vi "Test web service.vi"() -> ()   [LabVIEW 2012]
uses:
  Library/Shot data.ctl
panel:
  in  "Shot data":T1={"Shot number"=33, "Time"=timestamp(3410450400.259543 s since 1904-01-01), "Magnet ID"="sdqwde", "User"="sAXWCD", "Cell number"=1, "Requested field"=65.0, "Field direction"="UP", "Number of bank frames"=8, "Crowbar resistance, mOhm"=25.0, "Magnet resistance, mOhm"=35.0, "Charger voltage, kV"=9.0, "Frame voltage, kV"=10.0}
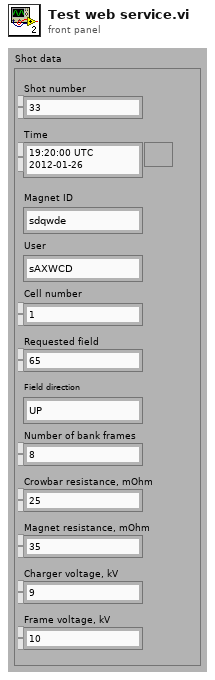
[diagram p1: front panel]
types:
  T1 = typedef "Shot data.ctl" = cluster{"Shot number":i32, "Time":timestamp, "Magnet ID":string, "User":string, "Cell number":i32, "Requested field":dbl, "Field direction":string, "Number of bank frames":i32, "Crowbar resistance, mOhm":dbl, "Magnet resistance, mOhm":dbl, "Charger voltage, kV":dbl, "Frame voltage, kV":dbl}
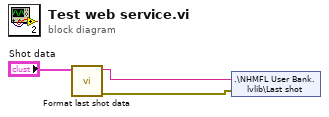
[diagram p0: block diagram]
diagram:
  n1 = call "Format last shot data.vi"("Shot data"="Shot data") -> ("error out"=w2:errorcluster, "Formated shot data"=w3:string)  [unwired: 7 in, 2 out]
  n2 = shared-variable ".\\NHMFL User Bank.lvlib\\Last shot"(w3, error in=w2) -> ()  [unwired: 1 out]
